vi "LogErrorEvent.vi"(8 "error in (no error)":errorcluster, 10 "ErrorEvent":errorcluster, 11 "EventLoggerData in":T1) -> (0 "error out":errorcluster, 3 "EventLoggerData out 3":T1)   [LabVIEW 2019, in "EventLogger.lvlib"]
uses:
  EventLogger.lvlib
  Cluster - EventLoggerData.ctl
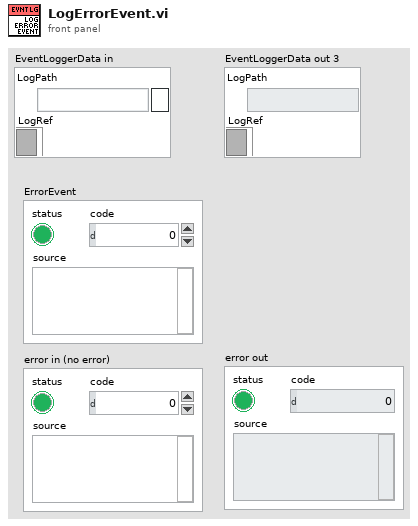
[diagram p1: front panel]
types:
  T1 = typedef "EventLogger.lvlib/Cluster - EventLoggerData.ctl" = cluster{"LogPath":path, "LogRef":refnum<file>}
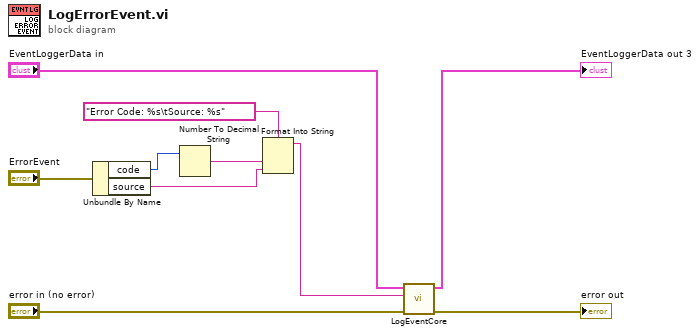
[diagram p0: block diagram]
diagram:
  n1 = Unbundle By Name("ErrorEvent") -> ("code"=w1:i32, "source"=w7:string)
  n2 = Number To Decimal String(number=w1) -> (decimal integer string=w8:string)  [unwired: 1 in]
  n3 = Format Into String(format string="Error Code: %s\tSource: %s", w8, w7) -> (resulting string=w2:string)  [unwired: 2 in, 1 out]
  n4 = call "LogEventCore.vi"("error in (no error)"="error in (no error)", "Event"=w2, "EventLoggerData in in"="EventLoggerData in") -> ("error out"=→"error out":errorcluster, "EventLoggerData out"=→"EventLoggerData out 3":T1)  [unwired: 7 in]
